vi "Read limit_x_up.vi"(8 "error in (no error)":errorcluster, 11 "PongPanel in":refnum<class "PongPanel.lvclass">) -> (0 "error out":errorcluster, 2 "limit_x_up":dbl, 3 "PongPanel out":refnum<class "PongPanel.lvclass">)   [LabVIEW 2019, in "RT_Game.lvlib" / "PongPanel.lvclass"]
uses:
  PongPanel.lvclass
  PongPanel.lvclass/PongPanel.ctl
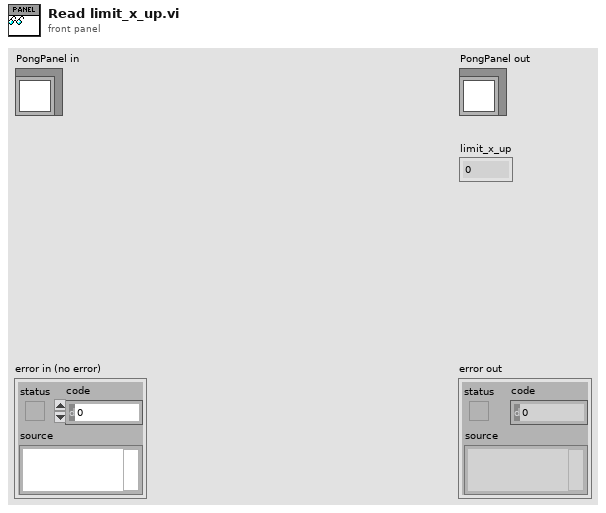
[diagram p1: front panel]
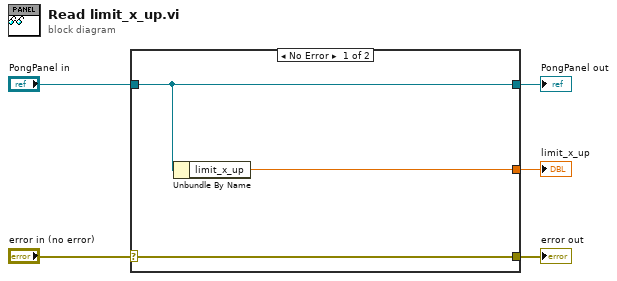
[diagram p0: block diagram]
diagram:
  n1 = case shown="No Error" "error in (no error)" {
    selector: "error in (no error)" -> [w8 w9]
    tunnel: [w8 w9] -> w4
    tunnel: [w7 w10] -> w2
    tunnel: "PongPanel in" -> [w7 w10]
    tunnel: [w6 _] -> w1
    frame No Error {
      n2 = Unbundle By Name(w7) -> ("limit_x_up"=w6:dbl)
    }
    frame Error {
    }
  }
  "error out" <- w4
  "PongPanel out" <- w2
  "limit_x_up" <- w1
